vi "_VIVIs.vi"() -> (3 "Array":refnum<vi>[](array[refnum]))   [LabVIEW 2017, in "tagdb-RefMgr Operations.lvlib"]
uses:
  tagdb-RefMgr Operations.lvlib
  VI_SetTitle.vi
  VI_Frontmost.vi
  VI_Closeable.vi
  VI_Resizable.vi
  VI_Minimizable.vi
  VI_ShowTitlebar.vi
  VI_ShowMenubar.vi
  VI_ShowToolbar.vi
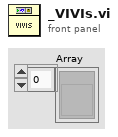
[diagram p1: front panel]
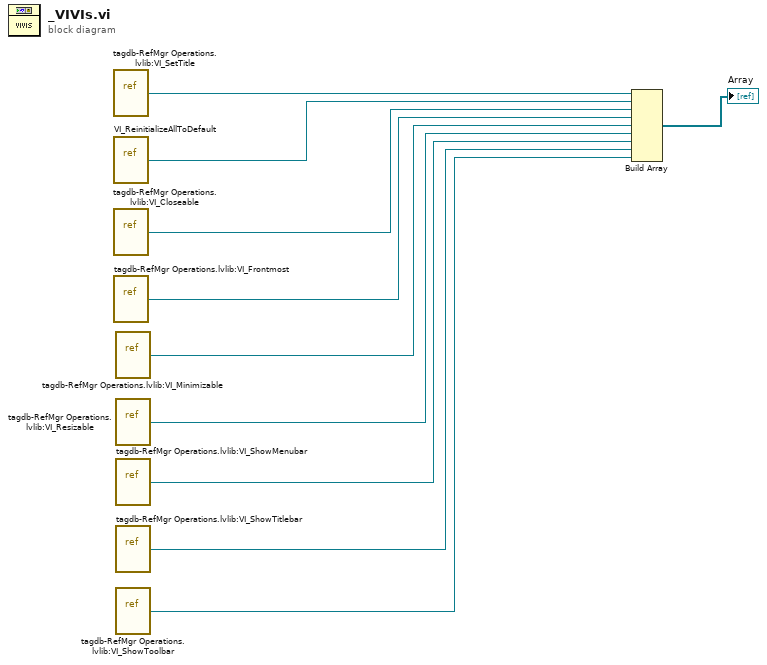
[diagram p0: block diagram]
diagram:
  n1 = vi-ref "tagdb-RefMgr Operations.lvlib:VI_SetTitle.vi"() -> (w8:refnum<vi>)
  n2 = vi-ref "VI_ReinitializeAllToDefault.vi"() -> (w10:refnum<vi>)
  n3 = vi-ref "tagdb-RefMgr Operations.lvlib:VI_Closeable.vi"() -> (w7:refnum<vi>)
  n4 = vi-ref "tagdb-RefMgr Operations.lvlib:VI_Frontmost.vi"() -> (w6:refnum<vi>)
  n5 = vi-ref "tagdb-RefMgr Operations.lvlib:VI_Minimizable.vi"() -> (w5:refnum<vi>)
  n6 = vi-ref "tagdb-RefMgr Operations.lvlib:VI_Resizable.vi"() -> (w4:refnum<vi>)
  n7 = vi-ref "tagdb-RefMgr Operations.lvlib:VI_ShowMenubar.vi"() -> (w3:refnum<vi>)
  n8 = vi-ref "tagdb-RefMgr Operations.lvlib:VI_ShowTitlebar.vi"() -> (w2:refnum<vi>)
  n9 = vi-ref "tagdb-RefMgr Operations.lvlib:VI_ShowToolbar.vi"() -> (w1:refnum<vi>)
  n10 = Build Array(w8, w10, w7, w6, w5, w4, w3, w2, w1) -> (→"Array":refnum<vi>[])
